vi "Get Request Queue.vi"(8 "error in (no error)":errorcluster, 11 "output_poller_queue in":refnum<class "output_poller_queue.lvclass">) -> (0 "error out":errorcluster, 2 "request_queue":refnum<queue>, 3 "output_poller_queue out":refnum<class "output_poller_queue.lvclass">)   [LabVIEW 2015, in "output_poller_queue.lvclass"]
uses:
  output_poller_queue.lvclass
  request/request.lvclass
  output_poller_queue.lvclass/output_poller_queue.ctl
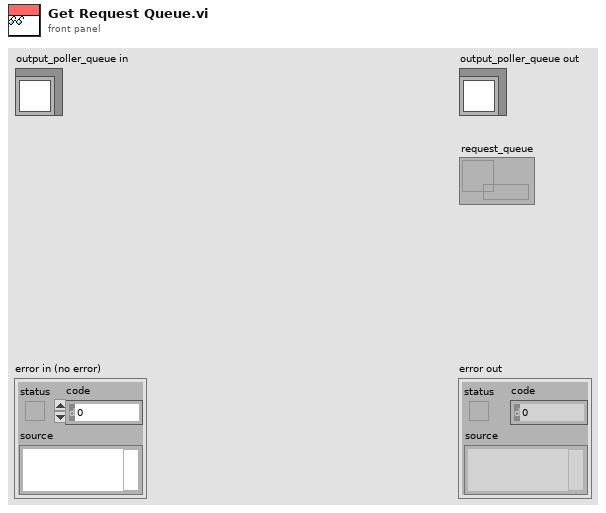
[diagram p1: front panel]
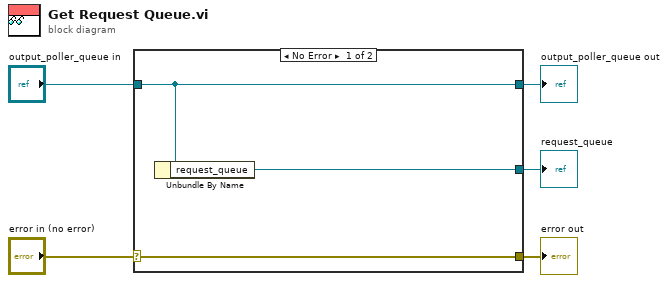
[diagram p0: block diagram]
diagram:
  n1 = case shown="No Error" "error in (no error)" {
    selector: "error in (no error)" -> [w8 w9]
    tunnel: [w8 w9] -> w4
    tunnel: [w7 w10] -> w2
    tunnel: "output_poller_queue in" -> [w7 w10]
    tunnel: [w6 _] -> w1
    frame No Error {
      n2 = Unbundle By Name(w7) -> ("request_queue"=w6:refnum<queue>)
    }
    frame Error {
    }
  }
  "error out" <- w4
  "output_poller_queue out" <- w2
  "request_queue" <- w1
